vi "Convert Packet String.vi"() -> ()   [LabVIEW 2017]
uses:
  Controls/Packet Data.ctl
panel:
  in  "String 2":string
  out "value":u32
  out "String":string
  out "reversed array":string[](array[string])
  in  "Number of bytes in packet":i32
  out "Array of nibbles":string[](array[string])
  in  "Buffer (hex)":string="13B5 0B00 0200 0000 2A00 0000 B0CF D03E 6FC1 B1BF 3561 333D 5F0E 1A3F 8FDD 2D3F E9FD C93E F23B 143E 0000 0400 0000 0000 0080 0000 0080 0000 0000 0000 0080 0000 0080 0000 0000 0000 80BF 0000 2222 2222 C2F9 B840 0000 0000 0000 0000 "
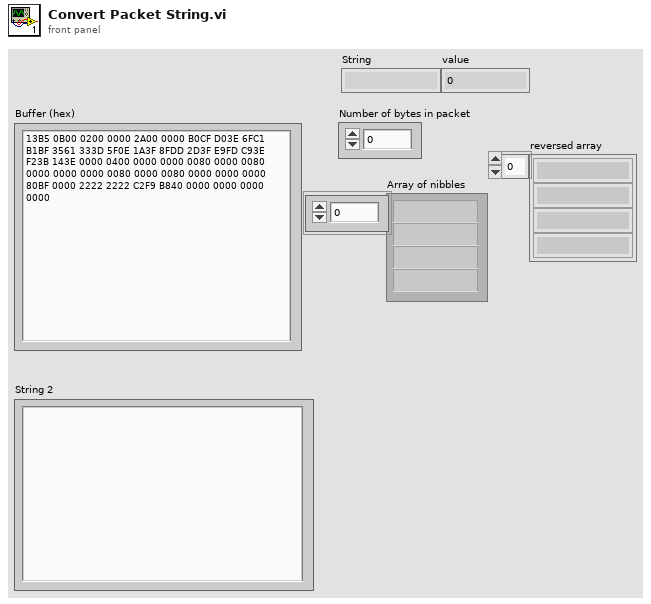
[diagram p1: front panel]
types:
  T1 = typedef "Packet Data.ctl" = cluster{"Frame Number (UINT32)":u32, "Number of Rigid Bodies (UINT32)":u32, "Timestamp (double float)":dbl}
  T2 = cluster{"Body ID (UINT32)":u32, "x (single float)":sgl, "y (single float)":sgl, "z (single float)":sgl, "qx (single float)":sgl, "qy (single float)":sgl, "qz (single float)":sgl, "qw (single float)":sgl, "Tracked 1 (UINT8)":u8, "Tracked 2 (UINT8)":u8}
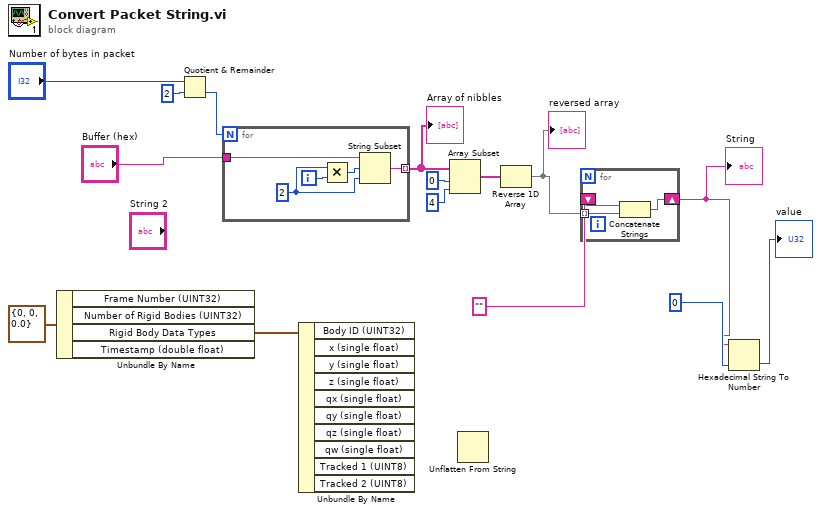
[diagram p0: block diagram]
diagram:
  n1 = Unbundle By Name(T1 {"Frame Number (UINT32)"=0, "Number of Rigid Bodies (UINT32)"=0, "Timestamp (double float)"=0.0} ("Data Types")) -> ("Rigid Body Data Types"=w1:T2)  [unwired: 3 out]
  n2 = Quotient & Remainder(x="Number of bytes in packet", y=2) -> (floor(x/y)=w8:i32)  [unwired: 1 out]
  n3 = for {
    N: w8 -> [_]
    tunnel: "Buffer (hex)" -> [w20]
    tunnel: [w19] -> w12 mode=indexing
    i -> [w18]
    w17 = 2
    n4 = Multiply(x=w17, y=w18) -> (x*y=w16:i32)
    n5 = String Subset(string=w20, offset (0)=w16, length (rest)=w17) -> (substring=w19:string)
  }
  "Array of nibbles" <- w12
  n6 = Unbundle By Name(w1) -> ()  [unwired: 10 out]
  n7 = Array Subset(array=w12, index=0, length=4) -> (w9:string[])
  n8 = Unflatten From String() -> ()  [unwired: 5 in, 3 out]
  n9 = Reverse 1D Array(array=w9) -> (reversed array=w7:string[])
  "reversed array" <- w7
  n10 = for {
    tunnel: w7 -> [w23] mode=indexing
    shift-right: [w21] -> w3
    shift-left: "" -> [w22]
    n11 = Concatenate Strings(w22, w23) -> (w21:string)
  }
  "String" <- w3
  n12 = Hexadecimal String To Number(string=w3, default (0uL)=u32 0) -> (number=→"value":u32)  [unwired: 1 in, 1 out]
